vi "StdObjectArray_write_and_unlock.vi"(8 "error in (no error)":errorcluster, 11 "StandardObjects":refnum<class "Standard.lvclass">[](array[class])) -> (0 "error out":errorcluster)   [LabVIEW 2017]
doc: "the VI writes and unlocks the StandardObjectsArray using a Queue"
uses:
  Classes/Standard/Standard.lvclass
  global variables.vi
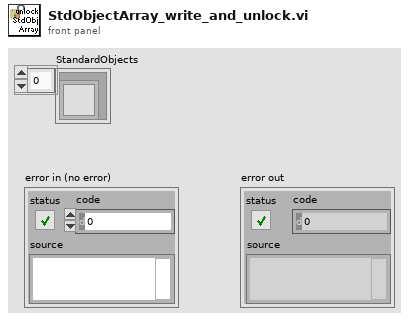
[diagram p1: front panel]
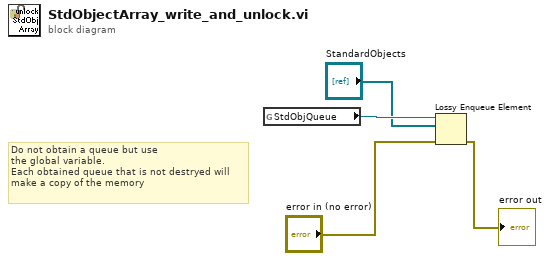
[diagram p0: block diagram]
diagram:
  # "Do not obtain a queue but use\nthe global variable.\nEach obtained queue that is not destryed will\nmake a copy of the memory"
  n1 = global read "global variables.vi" "StdObjQueue"() -> (w3:refnum<queue>)
  n2 = Lossy Enqueue Element(queue=w3, element="StandardObjects", error in (no error)="error in (no error)") -> (error out=→"error out":errorcluster)  [unwired: 3 out]
